vi "Get Protocol Classes List.vi"(8 "error in (no error)":errorcluster) -> (0 "error out":errorcluster, 3 "Class Lookup":variant)   [LabVIEW 2024, in "Instrument Addon Scripting API.lvlib"]
uses:
  Instrument Addon Scripting API.lvlib
  <vilib>/Utility/LVLibp/NI_PackedLibraryUtility.lvlib
  NationalInstruments.VeriStand
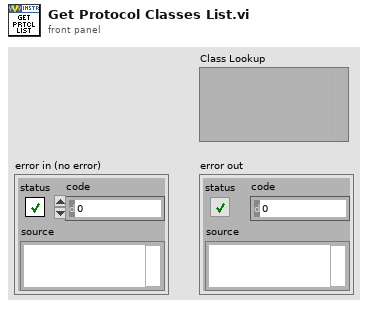
[diagram p1: front panel]
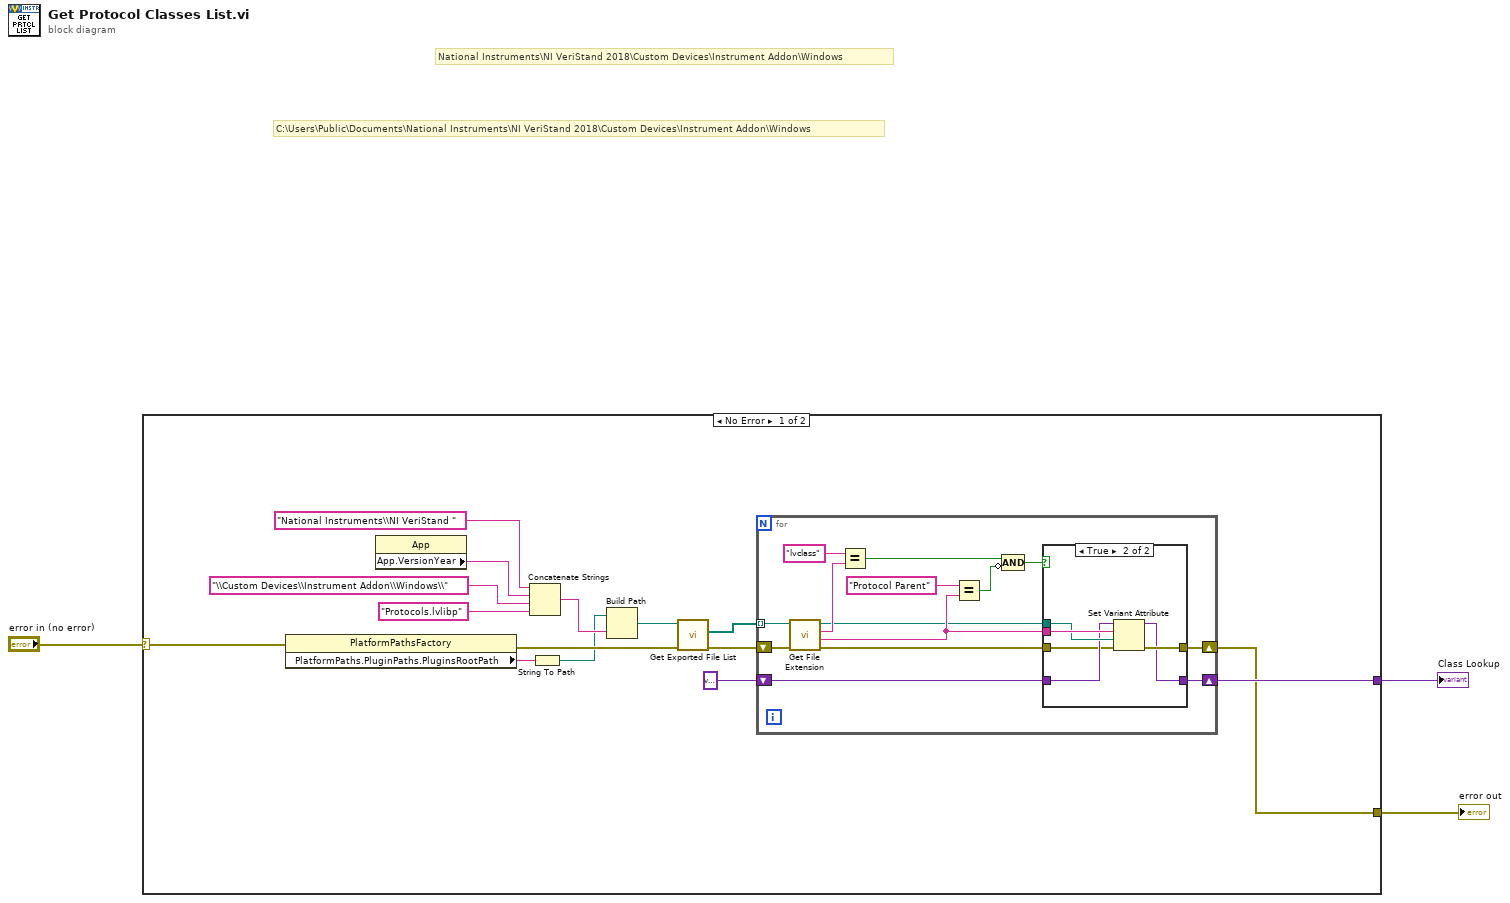
[diagram p0: block diagram]
diagram:
  # "National Instruments\\NI VeriStand 2018\\Custom Devices\\Instrument Addon\\Windows"
  # "C:\\Users\\Public\\Documents\\National Instruments\\NI VeriStand 2018\\Custom Devices\\Instrument Addon\\Windows"
  n1 = case shown="No Error" "error in (no error)" {
    selector: "error in (no error)" -> [w7 w41]
    tunnel: [w18 _] -> w3
    tunnel: [w17 w41] -> w2
    frame No Error {
      n2 = property class="PlatformPathsFactory"(error in=w7) -> (error out=w8:errorcluster, "PlatformPaths.PluginPaths.PluginsRootPath"=w6:string)  [unwired: 1 in, 1 out]
      n3 = property class="App"() -> ("App.VersionYear"=w4:string)  [unwired: 2 in, 2 out]
      n4 = Concatenate Strings("National Instruments\\NI VeriStand " ("string"), w4, "\\Custom Devices\\Instrument Addon\\Windows\\" ("string"), "Protocols.lvlibp" ("name or relative path")) -> (w16:string)
      n5 = String To Path(string=w6) -> (path=w5:path)
      n6 = Build Path(base path=w5, name or relative path=w16) -> (appended path=w9:path)
      n7 = call <vilib>:"Get Exported File List.vi"("error in (no error)"=w8, "packed library path"=w9) -> ("error out"=w11:errorcluster, "paths"=w10:path[])  [unwired: 7 in, 1 out]
      n8 = for {
        tunnel: w10 -> [w27] mode=indexing
        shift-right: [w21] -> w17
        shift-left: w11 -> [w28]
        shift-right: [w20] -> w18
        shift-left: variant ("variant") -> [w23]
        n9 = call <vilib>:"Get File Extension.vi"("error in (no error)"=w28, "file"=w27) -> ("error out"=w22:errorcluster, "filename without extension"=w25:string, "lowercase file extension"=w29:string, "dup file"=w24:path)  [unwired: 5 in, 1 out]
        n10 = Equal?(x="lvclass" ("string"), y=w29) -> (x = y?=w31:bool)
        n11 = Equal?(x="Protocol Parent", y=w25) -> (x = y?=w26:bool)
        n12 = Compound Arithmetic op=AND(w31, invert w26) -> (w19:bool)
        n13 = case shown="True" w19 {
          tunnel: w25 -> [_ w40]
          tunnel: w24 -> [_ w39]
          tunnel: w23 -> [w33 w38]
          tunnel: w22 -> [w34 w37]
          tunnel: [w34 w36] -> w21
          tunnel: [w33 w35] -> w20
          frame False {
          }
          frame True {
            n14 = Set Variant Attribute(Variant=w38, name=w40, value=w39, error in=w37) -> (Variant out=w35:variant, error out=w36:errorcluster)  [unwired: 1 out]
          }
        }
      }
    }
    frame Error {
    }
  }
  "Class Lookup" <- w3
  "error out" <- w2
